vi "Update State.vi"(8 "error in (no error)":errorcluster, 11 "SolarShutt in":refnum<class "SolarShutt.lvclass">) -> (0 "error out":errorcluster, 3 "SolarShutt out":refnum<class "SolarShutt.lvclass">)   [LabVIEW 2016]
uses:
  SolarShutt.lvclass
  Controls/Shutter States.ctl
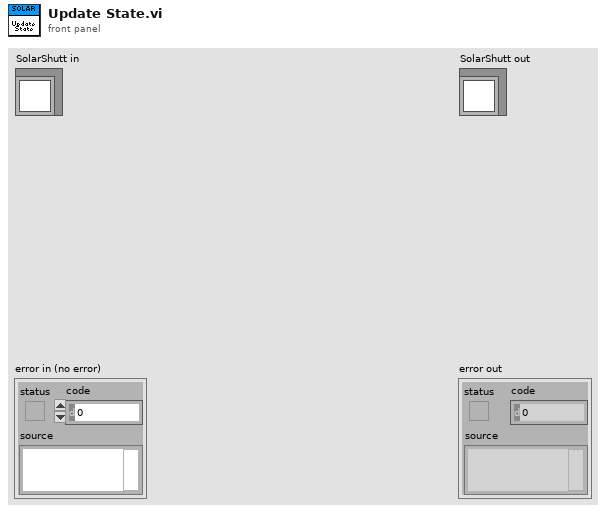
[diagram p1: front panel]
types:
  T1 = typedef "Shutter States.ctl" = enum16{"Open", "Close", "Wait", "Off", "Arm", "Idle"}
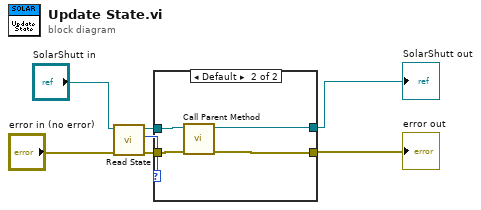
[diagram p0: block diagram]
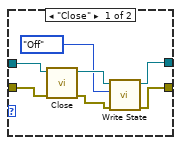
[diagram p2: hidden frame]
diagram:
  n1 = call-dynamic "Read State.vi"("error in (no error)"="error in (no error)", "Shutter in"="SolarShutt in") -> ("error out"=w3:errorcluster, "State"=w2:T1, "Shutter out"=w5:refnum<class "SolarShutt.lvclass">)  [unwired: 7 in]
  n2 = case shown="Default" w2 {
    tunnel: [w9 w18] -> w7
    tunnel: [w8 w17] -> w1
    tunnel: w5 -> [w14 w16]
    tunnel: w3 -> [w13 w15]
    frame "Close" {
      n3 = call-dynamic "Close.vi"("error in (no error)"=w13, "UniStableShutter in"=w14) -> ("error out"=w10:errorcluster, "UniStableShutter out"=w12:refnum<class "SolarShutt.lvclass">)  [unwired: 8 in]
      n4 = call-dynamic "Write State.vi"("error in (no error)"=w10, "Set"=Shutter_States."Off", "Shutter in"=w12) -> ("error out"=w9:errorcluster, "Shutter out"=w8:refnum<class "SolarShutt.lvclass">)  [unwired: 7 in]
    }
    frame Default {
      n5 = call-parent "Call Parent Method"("error in (no error)"=w15, "UniStableShutter in"=w16) -> ("error out"=w18:errorcluster, "UniStableShutter out"=w17:refnum<class "SolarShutt.lvclass">)  [unwired: 8 in]
    }
  }
  "error out" <- w7
  "SolarShutt out" <- w1
